vi "Organize Data by Sort Property.vi"(7 "Connection Refnum":T1, 8 "error in (no error)":errorcluster, 9 "Sort Property Name":string, 10 "Table":T2[](array[typedef]), 11 "Start Index":i32) -> (0 "error out":errorcluster, 1 "Property Value":string, 2 "Channel Data":dbl[](array[numeric]), 3 "End Index":i32)   [LabVIEW 2011]
uses:
  CGI SimpleStat Results.ctl
  SI.LIB/ODBC/SQL Controls/Connection Refnum.ctl
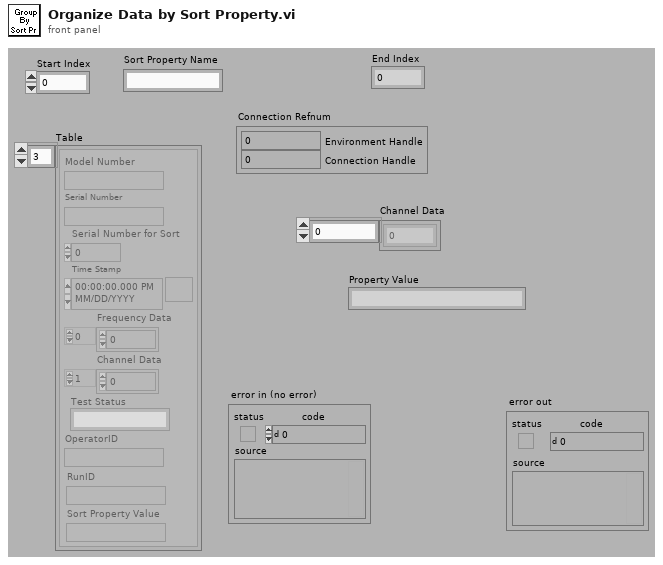
[diagram p1: front panel]
types:
  T1 = typedef "Connection Refnum.ctl" = cluster{"Environment Handle":i32, "Connection Handle":i32}
  T2 = typedef "CGI SimpleStat Results.ctl" = cluster{"Model Number":string, "Serial Number for Sort":i32, "Serial Number":string, "Time Stamp":timestamp, "Channel Data":dbl[], "Test Status":string, "OperatorID":string, "Frequency Data":dbl[], "RunID":string, "Sort Property Value":string}
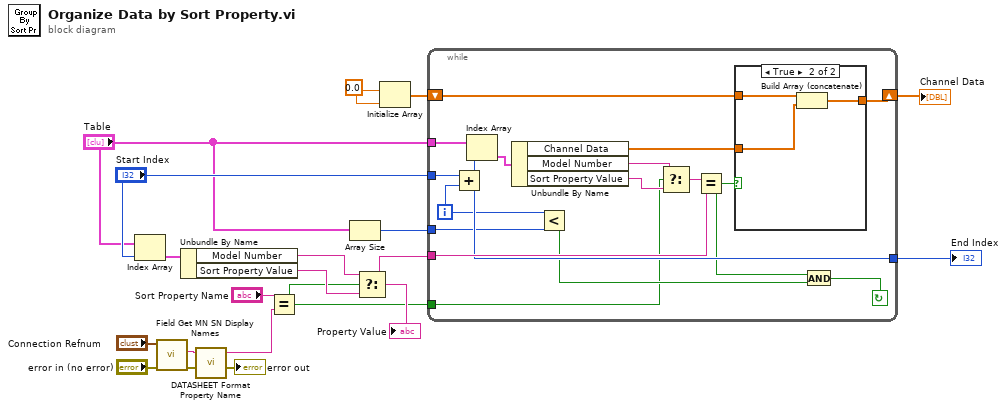
[diagram p0: block diagram]
diagram:
  w15 = 0.0
  n1 = Index Array(array="Table", index="Start Index") -> (element=w18:T2)
  n2 = call "Field Get MN SN Display Names.vi"("error in (no error)"="error in (no error)", "Connection Refnum"="Connection Refnum") -> ("error out"=→"error out":errorcluster, "Model Number Display Name"=w6:string)  [unwired: 8 out]
  n3 = Unbundle By Name(w18) -> ("Model Number"=w10:string, "Sort Property Value"=w8:string)
  n4 = call "DATASHEET Format Property Name.vi"("String with \\r or \\n"=w6) -> ("String without \\r or \\n"=w5:string)  [unwired: 4 out]
  n5 = Equal?(x="Sort Property Name", y=w5) -> (x = y?=w7:bool)
  n6 = Array Size(array="Table") -> (size(s)=w4:i32)
  n7 = Select(t=w10, s=w7, f=w8) -> (s? t:f=w9:string)
  "Property Value" <- w9
  n8 = Initialize Array(w15, w15) -> (w16:dbl[])
  n9 = while {
    tunnel: "Start Index" -> [w35]
    tunnel: "Table" -> [w34]
    shift-right: [w30] -> w14
    shift-left: w16 -> [w32]
    tunnel: w9 -> [w29]
    tunnel: [w28] -> w13
    tunnel: w4 -> [w24]
    tunnel: w7 -> [w19]
    i -> [w25]
    stop <- w26 continue-if-true
    n10 = Add(x=w35, y=w25) -> (x+y=w28:i32)
    n11 = Index Array(array=w34, index=w28) -> (element=w33:T2)
    n12 = Unbundle By Name(w33) -> ("Channel Data"=w31:dbl[], "Model Number"=w21:string, "Sort Property Value"=w20:string)
    n13 = Less?(x=w25, y=w24) -> (x < y?=w23:bool)
    n14 = Select(t=w21, s=w19, f=w20) -> (s? t:f=w22:string)
    n15 = Equal?(x=w22, y=w29) -> (x = y?=w27:bool)
    n16 = case shown="True" w27 {
      tunnel: w32 -> [w36 w39]
      tunnel: w31 -> [_ w38]
      tunnel: [w36 w37] -> w30
      frame False {
      }
      frame True {
        n17 = Build Array (concatenate)(w39, w38) -> (w37:dbl[])
      }
    }
    n18 = And(x=w27, y=w23) -> (x .and. y?=w26:bool)
  }
  "Channel Data" <- w14
  "End Index" <- w13
